vi "G#SubSubClass2_Create.vi"(0 "reference in":refnum<class "G#SubSubClass2.lvclass">, 5 "error in (no error)":errorcluster) -> (14 "reference out":refnum<class "G#SubSubClass2.lvclass">, 19 "error out":errorcluster)   [LabVIEW 2010, in "G#SubSubClass2.lvclass"]
doc: "Constructor."
uses:
  G#SubSubClass2.lvclass
  <vilib>/addons/_AddQ/G#Object/G#Object.lvclass
  G#SubClass2_class/G#SubClass2.lvclass
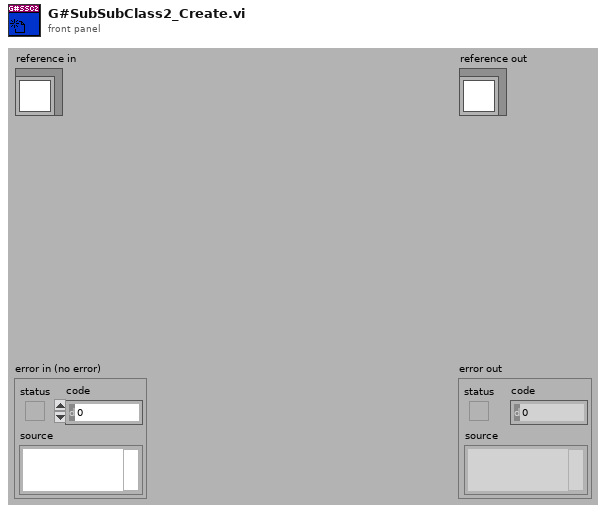
[diagram p1: front panel]
types:
  T1 = typedef "G#SubSubClass2.lvclass/ObjectAttributes.ctl" = cluster{"Base class":T2, "SubSubAttribute":dbl}
  T2 = typedef "G#SubClass2.lvclass/ObjectAttributes.ctl" = cluster{"Base class":T3, "SubAttribute":dbl}
  T3 = typedef "G#BaseClass2.lvclass/ObjectAttributes.ctl" = cluster{"Numeric":dbl, "Array":dbl[]}
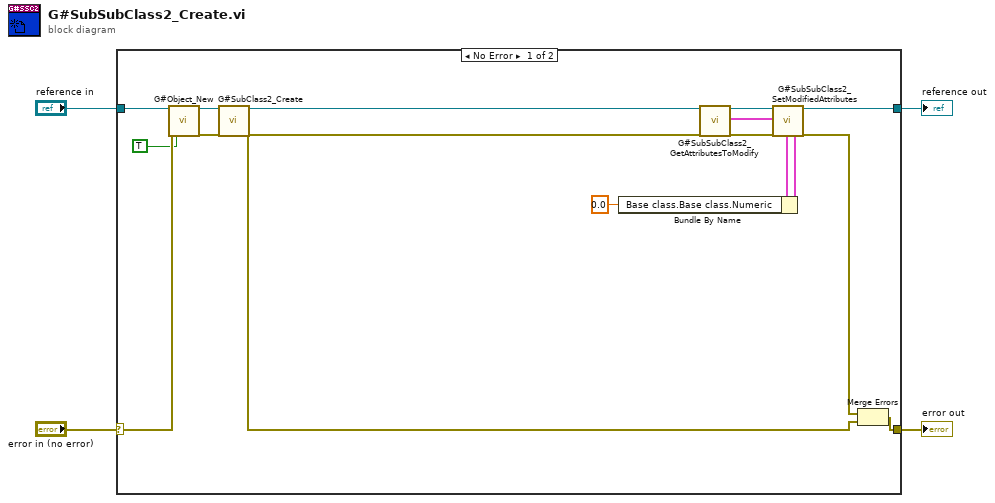
[diagram p0: block diagram]
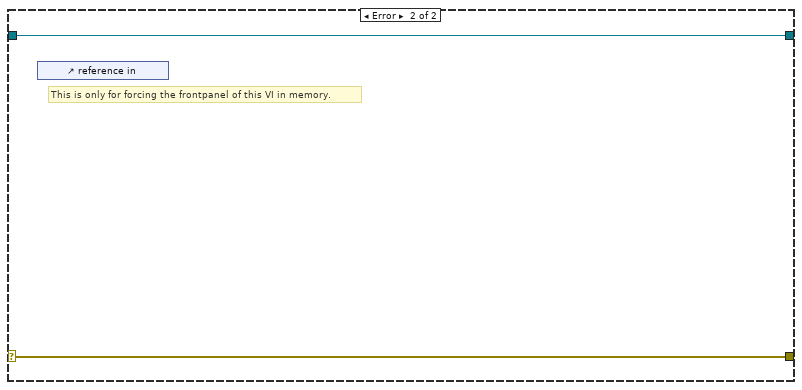
[diagram p2: hidden frame]
diagram:
  n1 = case shown="No Error" "error in (no error)" {
    selector: "error in (no error)" -> [w18 w21]
    tunnel: [w17 w21] -> w3
    tunnel: [w11 w20] -> w1
    tunnel: "reference in" -> [w19 w20]
    frame No Error {
      n2 = call <vilib>:"G#Object_New.vi"("reference in"=w19, "error in (no error)"=w18, "user counter (T)?"=TRUE ("User Counter")) -> ("reference out"=w16:refnum<class "G#SubSubClass2.lvclass">, "error out"=w15:errorcluster)  [unwired: 14 in, 1 out]
      n3 = call "G#SubClass2_Create.vi"("reference in"=w16, "error in (no error)"=w15) -> ("reference out"=w12:refnum<class "G#SubSubClass2.lvclass">, "error out"=w10:errorcluster)  [unwired: 16 in]
      n4 = call "G#SubSubClass2_GetAttributesToModify.vi"("reference in"=w12, "error in (no error)"=w10) -> ("reference out"=w13:refnum<class "G#SubSubClass2.lvclass">, "attributes"=w7:T1, "error out"=w9:errorcluster)  [unwired: 13 in, 2 out]
      n5 = Bundle By Name(cluster=w7, "Base class.Base class.Numeric"=0.0 ("Base class.Numeric")) -> (w6:T1)
      n6 = call "G#SubSubClass2_SetModifiedAttributes.vi"("reference in"=w13, "attributes"=w6, "error in (no error)"=w9) -> ("reference out"=w11:refnum<class "G#SubSubClass2.lvclass">, "error out"=w8:errorcluster)  [unwired: 15 in]
      n7 = Merge Errors(w8, w10) -> (w17:errorcluster)
    }
    frame Error {
      # "This is only for forcing the frontpanel of this VI in memory."
      n8 = control-ref of="reference in"() -> ()  [unwired: 1 out]
    }
  }
  "error out" <- w3
  "reference out" <- w1
